vi "Get Analog Value.vi"(8 "error in (no error)":errorcluster, 11 "Distance IR Bricklet in":refnum<class "Distance IR Bricklet.lvclass">) -> (0 "error out":errorcluster, 2 "Analog Value":u16, 3 "Distance IR Bricklet out":refnum<class "Distance IR Bricklet.lvclass">)   [LabVIEW 2011, in "Tinkerforge.lvlib" / "Distance IR Bricklet.lvclass"]
doc: "This VI returns the digital adc value from the illuminance sensor."
uses:
  Distance IR Bricklet.lvclass
  Device/Device.lvclass
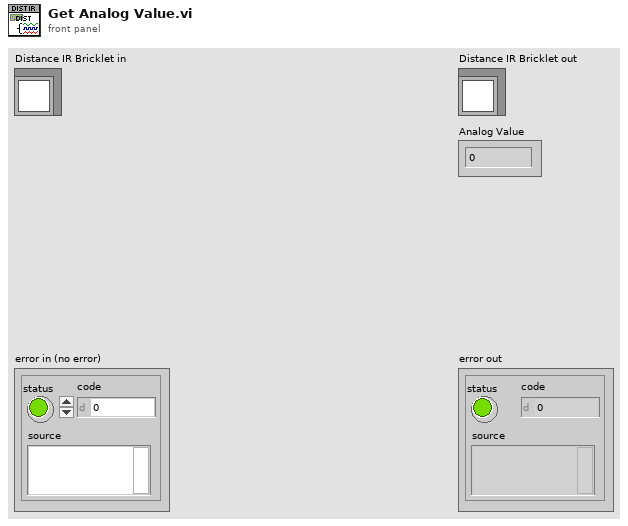
[diagram p1: front panel]
types:
  T1 = typedef "Tinkerforge.lvlib/IP Connection.lvclass/Answer.ctl" = cluster{"Request GUID":string, "Request Type":T2, "Sucessful":bool, "Data":variant, "Error":errorcluster}
  T2 = typedef "Tinkerforge.lvlib/IP Connection.lvclass/Request Type.ctl" = enum8{"Invalid", "Write"}
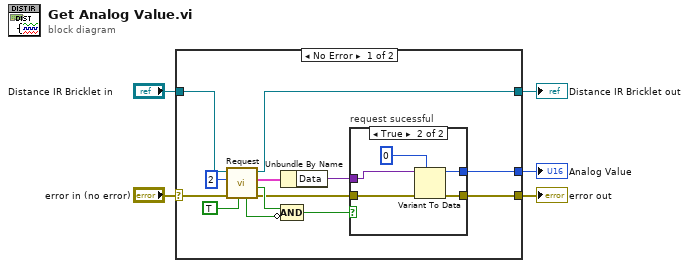
[diagram p0: block diagram]
diagram:
  n1 = case shown="No Error" "error in (no error)" {
    selector: "error in (no error)" -> [w18 w26]
    tunnel: [w7 w26] -> w4
    tunnel: [w16 w25] -> w2
    tunnel: "Distance IR Bricklet in" -> [w17 w25]
    tunnel: [w6 _] -> w1
    frame No Error {
      n2 = call "Request.vi"("Response"=TRUE, "error in (no error)"=w18, "Function ID"=u8 2, "Device in"=w17) -> ("error out"=w10:errorcluster, "Sucessful"=w12:bool, "Answer"=w9:T1, "Device out"=w16:refnum<class "Distance IR Bricklet.lvclass">, "timed out"=w13:bool)  [unwired: 3 in]
      n3 = Unbundle By Name(w9) -> ("Data"=w8:variant)
      n4 = Compound Arithmetic op=AND(w12, invert w13) -> (w11:bool)
      n5 = case "request sucessful" shown="True" w11 {
        tunnel: w10 -> [w19 w24]
        tunnel: w8 -> [_ w22]
        tunnel: [_ w21] -> w6
        tunnel: [w19 w20] -> w7
        frame False {
        }
        frame True {
          n6 = Variant To Data(error in=w24, type=u16 0, Variant=w22) -> (data=w21:u16, error out=w20:errorcluster)
        }
      }
    }
    frame Error {
    }
  }
  "error out" <- w4
  "Distance IR Bricklet out" <- w2
  "Analog Value" <- w1
